vi "client.set.vi"(8 "error in (no error)":errorcluster, 10 "Nominal Client":refnum<class "Nominal Client.lvclass">, 11 "Run in":refnum<class "Run.lvclass">) -> (0 "error out":errorcluster, 3 "Run out":refnum<class "Run.lvclass">)   [LabVIEW 2020, in "Run.lvclass"]
uses:
  Run.lvclass
  Run.lvclass/Run.ctl
  Nominal Client/Nominal Client.lvclass
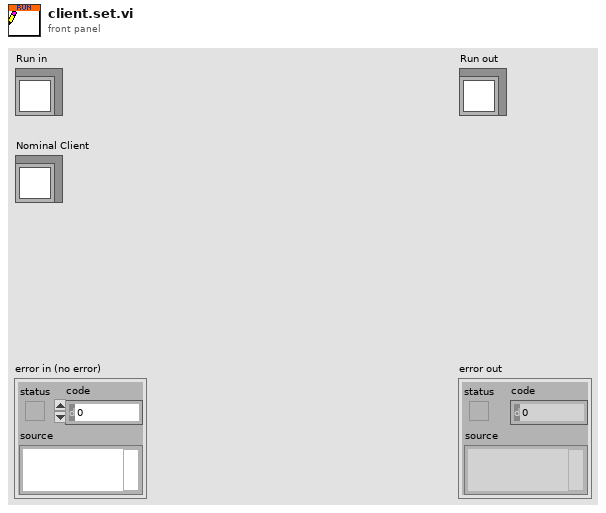
[diagram p1: front panel]
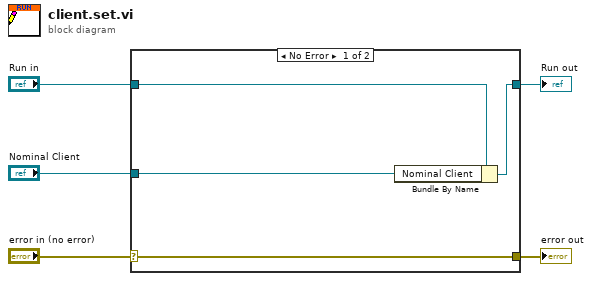
[diagram p0: block diagram]
diagram:
  n1 = case shown="No Error" "error in (no error)" {
    selector: "error in (no error)" -> [w9 w10]
    tunnel: [w9 w10] -> w4
    tunnel: [w7 w11] -> w2
    tunnel: "Run in" -> [w8 w11]
    tunnel: "Nominal Client" -> [w6 _]
    frame No Error {
      n2 = Bundle By Name(cluster=w8, "Nominal Client"=w6) -> (w7:refnum<class "Run.lvclass">)
    }
    frame Error {
    }
  }
  "error out" <- w4
  "Run out" <- w2
